vi "GUI main.vi"() -> ()   [LabVIEW 2020]
doc: "Use this template to build a producer/consumer design pattern with events to produce queue items. Use this design pattern instead of the User Interface Event Handler pattern for user interfaces when you want to execute code asynchronously in response to an event without slowing the user interface responsiveness."
uses:
  General PJVS driver/Type definitions/PJVS Type.ctl
  General PJVS driver/QPSsettings.ctl
  Measurement/Type definitions/Measuement properties.ctl
  Measurement/Type definitions/Measurement ID.ctl
  Measurement/Type definitions/Trigger mode.ctl
  General PJVS driver/Type definitions/PJVS Setup.ctl
  PJVS drivers/acsvcontrol-driver/build/ACSVcontrol-driver_0.2.0.0.llb/Timeouts.ctl
  PJVS drivers/JV modified NPL Bias source/DataSocketCluster external.ctl
  external libraries/AWG/AWG Session.ctl
  external libraries/AWG/AWG Type.ctl
  external libraries/AWG/CMI Clock Divider v2/CMI ckd2 Session.ctl
  external libraries/AWG/CMI Clock Divider v2/CMI ckd2 Source Mode.ctl
  external libraries/AWG/CMI Clock Divider v2/CMI ckd2 Divisor Mode.ctl
  external libraries/AWG/CMI Sync V3/CMI Sync V3 session.ctl
  external libraries/AWG/CMI Sync V3/Configure/CMI Sync V3 Reference Clock Source.ctl
  external libraries/AWG/CMI Sync V3/Configure/CMI Sync V3 HV input Range.ctl
  external libraries/AWG/CMI Sync V3/Configure/CMI Sync V3 Trigger Input Level.ctl
  external libraries/AWG/CMI Sync V3/Configure/CMI Sync V3 Channel 1 Mode.ctl
  external libraries/AWG/CMI Sync V3/Configure/CMI Sync V3 Channel Output Levels.ctl
  external libraries/AWG/CMI Sync V3/Configure/CMI Sync V3 Channel 2 Mode.ctl
  external libraries/AWG/CMI Sync V3/Configure/CMI Sync V3 Channel 3 Mode.ctl
  external libraries/AWG/CMI Sync V3/Configure/CMI Sync V3 Channel 1 Divisor Entry Mode.ctl
  external libraries/externals needed for AWG/ADC Trig Config.ctl
  external libraries/externals needed for AWG/ADC Trig Mode Source.ctl
  external libraries/externals needed for AWG/ADC Trig Coupling.ctl
  external libraries/externals needed for AWG/ADC Trig Slope.ctl
  external libraries/AWG/RaS HMF2500/HMF2500 Config.ctl
  <vilib>/Utility/error.llb/DialogType.ctl
  <vilib>/Utility/error.llb/Error Cluster From Error Code.vi
  <vilib>/ErrorRing/Error Ring.xnode
  external libraries/TWM client.lvlibp
  external libraries/varilib/varilib.lvlib
  PJVS drivers/acsvcontrol-driver/build/ACSVcontrol-driver_0.2.0.0.llb/ACSVcontrol-driver.lvlib
  external libraries/AWG/AWG.lvlib
  external libraries/AWG/CMI Sync V3/CMI Sync Unit V3.lvlib
panel:
  out "Measurement status":string
  in  "Setup awg":bool
  out "qps settings":T1={"TWM pipe name"="\\\\.\\pipe\\TWM:server", "meas"={"Measurement ID"=enum."1", "Description"="3 phase, 3 ADC, 1 PJVS", "Switching matrix M"=[], "Signal frequency  (Hz)"=50.0, "Signal amplitudes (V)"=[], "PRs (s)"=1.0, "PRe (s)"=10.0, "MRs (s)"=0.0, "MRe (s)"=0.0, "Set PJVS frequency (Hz)"=50.0, "PJVS reference voltages (1 period, V)"=[], "Requiested PJVS steps"=10, "Sampling f (Hz)"=0.0, "Trigger mode"=enum."Trigger every MX switch", "Timing matrix (periods)"=[], "Record length (multiples of M)"=1, "Calculated"={"Triggers to next path (line of sequence)"=[], "Record samples"=0, "Sample indexes of switches"=[], "PRs (samples)"=0, "PRe (samples)"=0, "MRs (samples)"=0, "MRe (samples)"=0, "Trigger frequency  (Hz)"=50.0, "Measurement druation (s)"=0.0}}, "PJVS setup"={"PJVS type"=enum."AC-supraVOLTcontrol", "Status Refnum"=refnum, "AC-supraVOLTcontrol"={"IP address:port (0.0.0.0:0000)"="0.0.0.0:0000", "Timeouts"={"TCP Read & Write (ms)"=7000, "Sensors readout"=5000, "PJVS setup"=10000, "Nullmeter readout"=5000, "Multiplexer setup"=3000, "57XX setup"=15000, "Generator setup"=5000, "Synthesizer setup"=3000, "Sampler readout"=10000}, "Simulation mode"=FALSE, "Debug mode"=FALSE}, "NPL bias source"={"DataSocketCluster"={"Server Machine"="CZC105BD8M", "Client Machine"="localhost", "Data"="P2", "TimeStamp"=0.0, "Count"=1, "Target Process"="General Server"}}}, "awg"={"type"=enum."Agilent 331xxA to 332xxA", "VISA"="", "enable 10MHz ref"=FALSE, "cmi ckd2"={"VISA"="", "clock source"=enum."Auto", "manual ref clk"=FALSE, "ref clock [Hz]"=0.0, "div mode"=enum."Set divisor directly"}, "cmi sync v3"={"VISA"="", "baud rate [bd/s]"=115200, "source"=enum."Auto", "hv range"=enum."1kV", "fsrc is fixed"=FALSE, "fsrc [Hz]"=10000000.0, "freq integ [s]"=1.0, "freq filter"=5, "trig level"=enum."TTL 5V", "chn1 mode"=enum."Source divider", "chn1 level"=enum."Positive 5V", "chn2 mode"=enum."Source divider", "chn2 level"=enum."Positive 5V", "chn2 div"=1, "chn3 mode"=enum."Chn 1 Active", "chn3 level"=enum."Positive 5V", "chn1 div entry"=enum."Calculate nearest divisor from measured fx", "chn1 dev limit [%]"=1.0, "chn1 check dev"=FALSE}, "trigger"={"source"=enum."Immediate", "level [V]"=0.0, "coupling"=enum."DC", "slope"=enum."POS"}, "HMF2500 cfg"={"Baud Rate"=9600, "Parity"=0, "Data Bits"=8, "Flow Control"=4}}, "Measurement status Ref"=refnum, "TWM status Ref"=refnum, "Abort Ref"=refnum} {"awg"."HMF2500 cfg"."Flow Control" items=["None", "XON/XOFF", "RTS/CTS", "XON/XOFF & RTS/CTS", "DTR/DSR", "XON/XOFF & DTR/DSR"]; "awg"."HMF2500 cfg"."Data Bits" items=["7"=7, "8"=8]; "awg"."HMF2500 cfg"."Parity" items=["None", "Odd", "Even", "Mark", "Space"]; "awg"."HMF2500 cfg"."Baud Rate" items=["300"=300, "600"=600, "1200"=1200, "2400"=2400, "4800"=4800, "9600"=9600, "19200"=19200]; "awg"."cmi sync v3"."chn2 div" min=1 max=100000000 step=1; "awg"."cmi sync v3"."fsrc [Hz]" format="%_8p"; "PJVS setup"."NPL bias source"."DataSocketCluster"."TimeStamp" format="%.2f"; "meas"."Calculated"."Trigger frequency  (Hz)" format="%#_6p"; "meas"."Record length (multiples of M)" min=1 step=1; "meas"."PJVS reference voltages (1 period, V)" format="%.9g"; "meas"."MRe (s)" format="%#_4p"; "meas"."MRs (s)" format="%#_4p"; "meas"."PRe (s)" format="%#.4p"; "meas"."PRs (s)" format="%#_4p"}
  in  "Measure":bool
  out "gui_unlock_for_measure":refnum<vi>[](array[refnum])
  out "gui_to_lock":refnum<vi>[](array[refnum])
  out "Measurement description":string
  in  "Setup meas":bool
  in  "Abort":bool
  out "PJVS status":string
  out "TWM Status":string
  out "PJVS":T6
  in  "Test TWM":bool
  in  "TWM pipe name":string="\\\\.\\pipe\\TWM:server"
  in  "About":bool
  in  "Setup pjvs":bool
  in  "Quit":bool
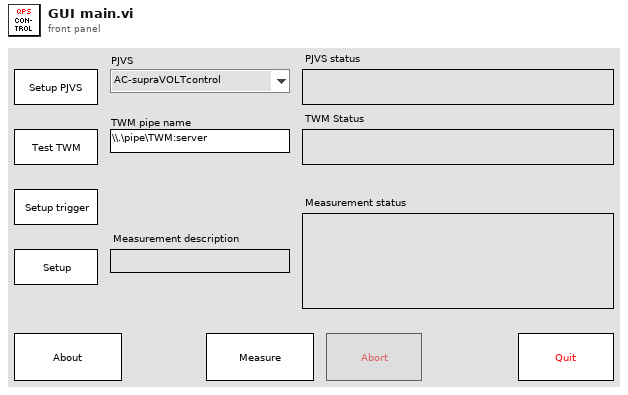
[diagram p1: front panel]
types:
  T1 = typedef "QPSsettings.ctl" = cluster{"TWM pipe name":string, "meas":T2, "PJVS setup":T5, "awg":T9, "Measurement status Ref":refnum<vi>, "TWM status Ref":refnum<vi>, "Abort Ref":refnum<vi>}
  T2 = typedef "Measuement properties.ctl" = cluster{"Measurement ID":T3, "Description":string, "Switching matrix M":u32[][], "Signal frequency  (Hz)":dbl, "Signal amplitudes (V)":dbl[], "PRs (s)":dbl, "PRe (s)":dbl, "MRs (s)":dbl, "MRe (s)":dbl, "Set PJVS frequency (Hz)":dbl, "PJVS reference voltages (1 period, V)":dbl[], "Requiested PJVS steps":u32, "Sampling f (Hz)":dbl, "Trigger mode":T4, "Timing matrix (periods)":i32[], "Record length (multiples of M)":u32, "Calculated":cluster{"Triggers to next path (line of sequence)":u32[], "Record samples":u32, "Sample indexes of switches":u32[], "PRs (samples)":i32, "PRe (samples)":i32, "MRs (samples)":i32, "MRe (samples)":i32, "Trigger frequency  (Hz)":dbl, "Measurement druation (s)":dbl}}
  T3 = typedef "Measurement ID.ctl" = enum16{"M", "1", "2", "3"}
  T4 = typedef "Trigger mode.ctl" = enum16{"Trigger every MX switch", "Trigger every sample"}
  T5 = typedef "PJVS Setup.ctl" = cluster{"PJVS type":T6, "Status Refnum":refnum<vi>, "AC-supraVOLTcontrol":cluster{"IP address:port (0.0.0.0:0000)":string, "Timeouts":T7, "Simulation mode":bool, "Debug mode":bool}, "NPL bias source":cluster{"DataSocketCluster":T8}}
  T6 = typedef "PJVS Type.ctl" = enum16{"AC-supraVOLTcontrol", "JV modified NPL bias control"}
  T7 = typedef "ACSVcontrol-driver.lvlib/Timeouts.ctl" = cluster{"TCP Read & Write (ms)":i32, "Sensors readout":i32, "PJVS setup":i32, "Nullmeter readout":i32, "Multiplexer setup":i32, "57XX setup":i32, "Generator setup":i32, "Synthesizer setup":i32, "Sampler readout":i32}
  T8 = typedef "DataSocketCluster external.ctl" = cluster{"Server Machine":string, "Client Machine":string, "Data":string, "TimeStamp":dbl, "Count":i32, "Target Process":string}
  T9 = typedef "AWG.lvlib/AWG Session.ctl" = cluster{"type":T10, "VISA":refnum<visa-resource-name>, "enable 10MHz ref":bool, "cmi ckd2":T11, "cmi sync v3":T14, "trigger":T23, "HMF2500 cfg":T27}
  T10 = typedef "AWG.lvlib/AWG Type.ctl" = enum16{"Agilent 331xxA to 332xxA", "Agilent 335xxA to 336xxA", "Tektronix AFG3101C", "R&S HMF25xx", "CMI Clock Divider v2", "CMI Sync Unit V3", "dummy"}
  T11 = typedef "AWG.lvlib/CMI ckd2 Session.ctl" = cluster{"VISA":refnum<visa-resource-name>, "clock source":T12, "manual ref clk":bool, "ref clock [Hz]":dbl, "div mode":T13}
  T12 = typedef "AWG.lvlib/CMI ckd2 Source Mode.ctl" = enum16{"Auto", "LF clock", "HF clock", "Internal"}
  T13 = typedef "AWG.lvlib/CMI ckd2 Divisor Mode.ctl" = enum16{"Set divisor directly", "Set divisor by frequency"}
  T14 = typedef "AWG.lvlib/CMI Sync Unit V3.lvlib/CMI Sync V3 session.ctl" = cluster{"VISA":refnum<visa-resource-name>, "baud rate [bd/s]":i32, "source":T15, "hv range":T16, "fsrc is fixed":bool, "fsrc [Hz]":dbl, "freq integ [s]":dbl, "freq filter":i32, "trig level":T17, "chn1 mode":T18, "chn1 level":T19, "chn2 mode":T20, "chn2 level":T19, "chn2 div":i32, "chn3 mode":T21, "chn3 level":T19, "chn1 div entry":T22, "chn1 dev limit [%]":dbl, "chn1 check dev":bool}
  T15 = typedef "AWG.lvlib/CMI Sync Unit V3.lvlib/CMI Sync V3 Reference Clock Source.ctl" = enum16{"Auto", "Internal", "Logic", "Sine", "HV"}
  T16 = typedef "AWG.lvlib/CMI Sync Unit V3.lvlib/CMI Sync V3 HV input Range.ctl" = enum16{"10V", "60V", "250V", "1kV"}
  T17 = typedef "AWG.lvlib/CMI Sync Unit V3.lvlib/CMI Sync V3 Trigger Input Level.ctl" = enum16{"LVCMOS 3V3", "TTL 5V"}
  T18 = typedef "AWG.lvlib/CMI Sync Unit V3.lvlib/CMI Sync V3 Channel 1 Mode.ctl" = enum16{"Source divider", "DDS absolute", "DDS ratio", "DDS ratio M/N"}
  T19 = typedef "AWG.lvlib/CMI Sync Unit V3.lvlib/CMI Sync V3 Channel Output Levels.ctl" = enum16{"Positive 3V3", "Negative 3V3", "Positive 5V", "Negative 5V"}
  T20 = typedef "AWG.lvlib/CMI Sync Unit V3.lvlib/CMI Sync V3 Channel 2 Mode.ctl" = enum16{"Source divider", "Chn 1 divide"}
  T21 = typedef "AWG.lvlib/CMI Sync Unit V3.lvlib/CMI Sync V3 Channel 3 Mode.ctl" = enum16{"Chn 1 Active", "Chn 2 Active", "Chn 1 Trigger", "Chn 2 Trigger", "Gate", "PPS", "10MHz"}
  T22 = typedef "AWG.lvlib/CMI Sync Unit V3.lvlib/CMI Sync V3 Channel 1 Divisor Entry Mode.ctl" = enum16{"Set divisor directly", "Calculate nearest divisor from measured fx"}
  T23 = typedef "ADC Trig Config.ctl" = cluster{"source":T24, "level [V]":dbl, "coupling":T25, "slope":T26}
  T24 = typedef "ADC Trig Mode Source.ctl" = enum16{"Immediate", "External", "Level"}
  T25 = typedef "ADC Trig Coupling.ctl" = enum16{"DC", "AC"}
  T26 = typedef "ADC Trig Slope.ctl" = enum16{"POS", "NEG"}
  T27 = typedef "AWG.lvlib/HMF2500 Config.ctl" = cluster{"Baud Rate":u32, "Parity":u16, "Data Bits":u16, "Flow Control":u16}
  T28 = typedef "DialogType.ctl" = u16
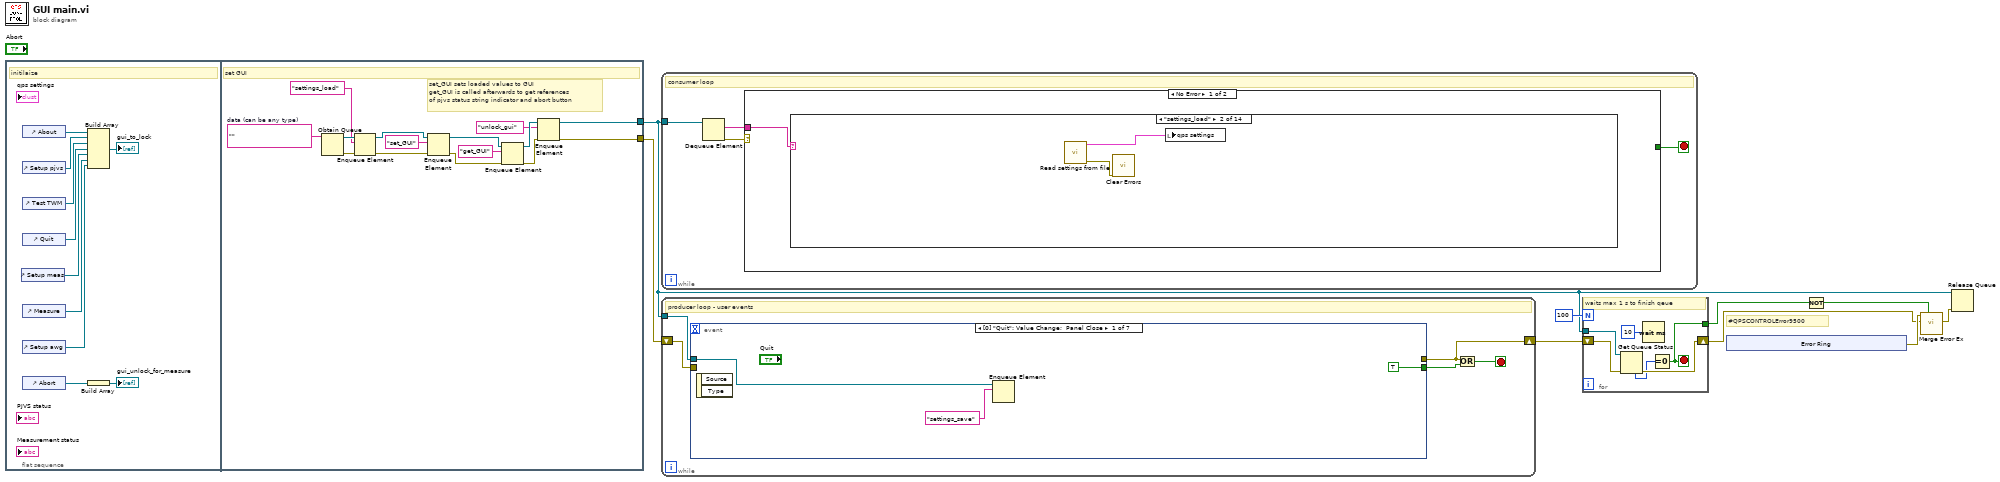
[diagram p0: block diagram]
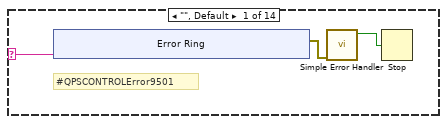
[diagram p2: hidden frame]
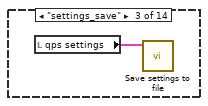
[diagram p3: hidden frame]
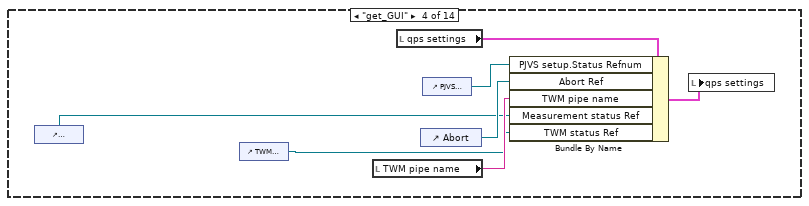
[diagram p4: hidden frame]
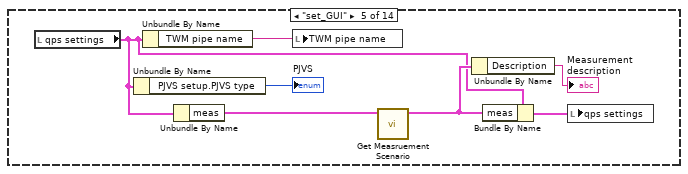
[diagram p5: hidden frame]
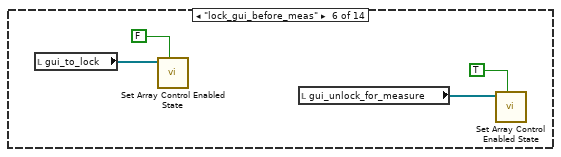
[diagram p6: hidden frame]
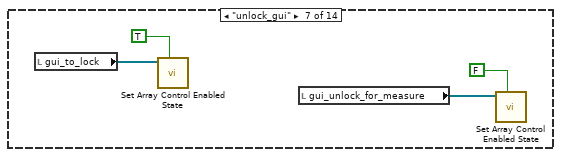
[diagram p7: hidden frame]
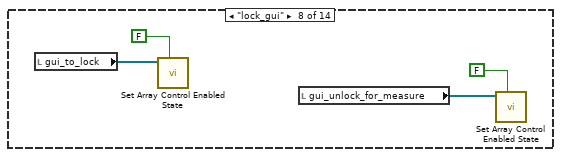
[diagram p8: hidden frame]
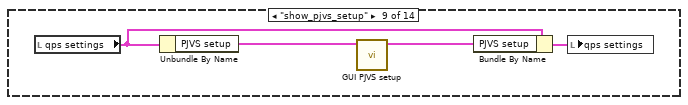
[diagram p9: hidden frame]
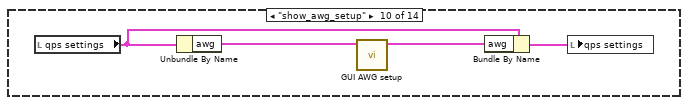
[diagram p10: hidden frame]
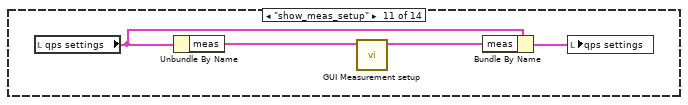
[diagram p11: hidden frame]
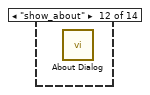
[diagram p12: hidden frame]
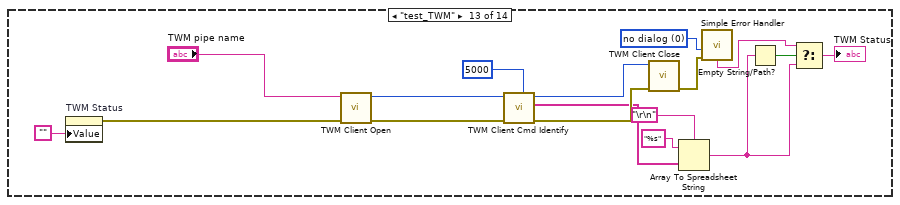
[diagram p13: hidden frame]
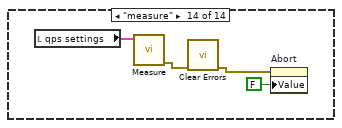
[diagram p14: hidden frame]
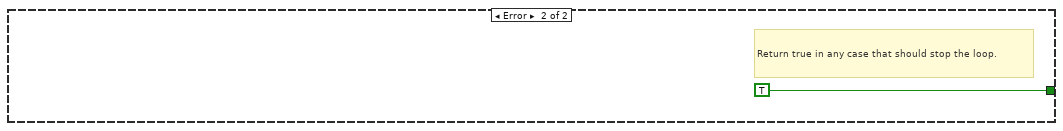
[diagram p15: hidden frame]
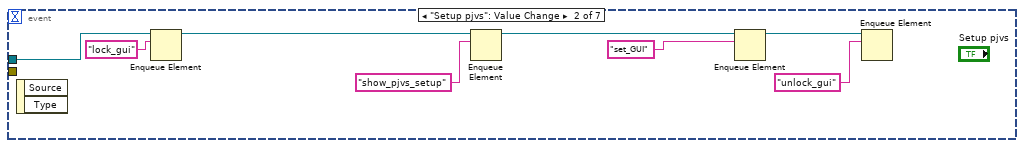
[diagram p16: hidden frame]
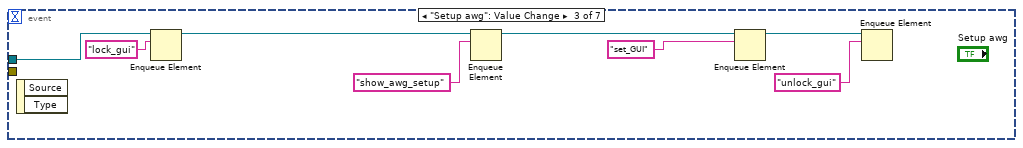
[diagram p17: hidden frame]
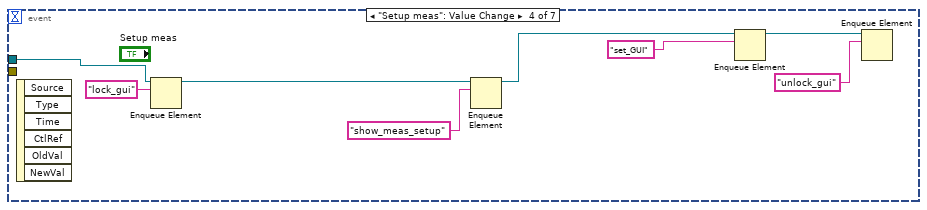
[diagram p18: hidden frame]
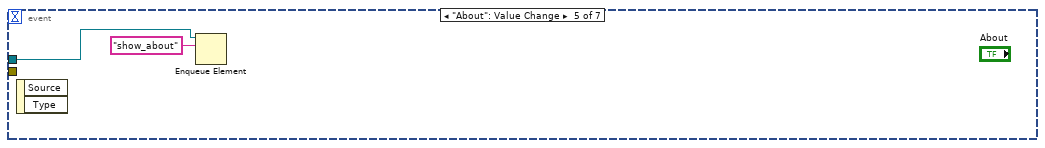
[diagram p19: hidden frame]
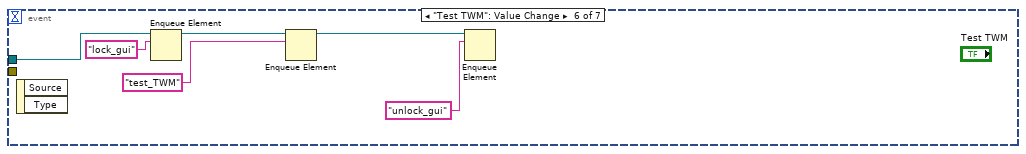
[diagram p20: hidden frame]
diagram:
  # "#QPSCONTROLError9500"
  n1 = flat-sequence {
    tunnel: [w24] -> w3
    tunnel: [w21] -> w9
    frame #0 {
      # "initilaize"
      n2 = control-ref of="Setup meas"() -> (w16:refnum<vi>)
      n3 = control-ref of="About"() -> (w12:refnum<vi>)
      n4 = control-ref of="Setup pjvs"() -> (w13:refnum<vi>)
      n5 = control-ref of="Test TWM"() -> (w14:refnum<vi>)
      n6 = control-ref of="Quit"() -> (w15:refnum<vi>)
      n7 = control-ref of="Measure"() -> (w11:refnum<vi>)
      n8 = control-ref of="Setup awg"() -> (w10:refnum<vi>)
      n9 = control-ref of="Abort"() -> (w17:refnum<vi>)
      n10 = Build Array(w12, w13, w14, w15, w16, w11, w10) -> (→"gui_to_lock":refnum<vi>[])
      n11 = Build Array(w17) -> (→"gui_unlock_for_measure":refnum<vi>[])
    }
    frame #1 {
      w34 = ""  # data (can be any type)
      # "set_GUI sets loaded values to GUI\nget_GUI is called afterwards to get references\nof pjvs status string indicator and abort button"
      # "set GUI"
      n12 = Obtain Queue(element data type=w34) -> (queue out=w33:refnum<queue>, error out=w32:errorcluster)  [unwired: 4 in, 1 out]
      n13 = Enqueue Element(queue=w33, element="settings_load", error in (no error)=w32) -> (queue out=w26:refnum<queue>, error out=w29:errorcluster)  [unwired: 1 in, 1 out]
      n14 = Enqueue Element(queue=w26, element="set_GUI", error in (no error)=w29) -> (queue out=w27:refnum<queue>, error out=w28:errorcluster)  [unwired: 1 in, 1 out]
      n15 = Enqueue Element(queue=w27, element="get_GUI", error in (no error)=w28) -> (queue out=w22:refnum<queue>, error out=w23:errorcluster)  [unwired: 1 in, 1 out]
      n16 = Enqueue Element(queue=w22, element="unlock_gui", error in (no error)=w23) -> (queue out=w24:refnum<queue>, error out=w21:errorcluster)  [unwired: 1 in, 1 out]
    }
  }
  n17 = while {
    tunnel: w3 -> [w38]
    stop <- w35 stop-if-true
    # "consumer loop"
    n18 = Dequeue Element(queue=w38) -> (element=w36:string, error out=w37:errorcluster)  [unwired: 2 in, 2 out]
    n19 = case shown="No Error" w37 {
      tunnel: w36 -> [w39 _]
      tunnel: [_ TRUE] -> w35
      frame No Error {
        n20 = case shown="\"settings_load\"" w39 {
          selector: w39 -> [w40 _ _ _ _ _ _ _ _ _ _ _ _ _]
          frame "", Default {
            # "#QPSCONTROLError9501"
            n21 = xnode "Error Ring"("parameter 0"=w40) -> ("error out"=w42:errorcluster)
            n22 = call <vilib>:"Simple Error Handler.vi"("error in (no error)"=w42) -> ("error?"=w41:bool)  [unwired: 4 in, 4 out]
            n23 = Stop(stop? (T)=w41) -> ()
          }
          frame "settings_load" {
            n24 = call "Read settings from file.vi"() -> ("error out"=w50:errorcluster, "QPS settings out"=w51:T1)  [unwired: 10 in]
            n25 = call <vilib>:"Clear Errors.vi"("error in (no error)"=w50) -> ()  [unwired: 5 in, 2 out]
            n26 = local write "qps settings"(w51) -> ()
          }
          frame "settings_save" {
            n27 = local read "qps settings"() -> (w52:T1)
            n28 = call "Save settings to file.vi"("QPS settings"=w52) -> ()  [unwired: 10 in, 1 out]
          }
          frame "get_GUI" {
            n29 = control-ref of="Measurement status"() -> (w54:refnum<vi>)
            n30 = control-ref of="TWM Status"() -> (w53:refnum<vi>)
            n31 = local read "TWM pipe name"() -> (w55:string)
            n32 = local read "qps settings"() -> (w59:T1)
            n33 = control-ref of="Abort"() -> (w57:refnum<vi>)
            n34 = control-ref of="PJVS status"() -> (w56:refnum<vi>)
            n35 = Bundle By Name(cluster=w59, "PJVS setup.Status Refnum"=w56, "Abort Ref"=w57, "TWM pipe name"=w55, "Measurement status Ref"=w54, "TWM status Ref"=w53) -> (w58:T1)
            n36 = local write "qps settings"(w58) -> ()
          }
          frame "set_GUI" {
            n37 = local read "qps settings"() -> (w61:T1)
            n38 = Unbundle By Name(w61) -> ("PJVS setup.PJVS type"=→"PJVS":T6)
            n39 = Unbundle By Name(w61) -> ("TWM pipe name"=w60:string)
            n40 = Unbundle By Name(w61) -> ("meas"=w64:T2)
            n41 = local write "TWM pipe name"(w60) -> ()
            n42 = call "Get Measruement Scenario.vi"("Measurement properties"=w64) -> ("Measurement properties out"=w63:T2)  [unwired: 10 in]
            n43 = Unbundle By Name(w63) -> ("Description"=→"Measurement description":string)
            n44 = Bundle By Name(cluster=w61, "meas"=w63) -> (w62:T1)
            n45 = local write "qps settings"(w62) -> ()
          }
          frame "lock_gui_before_meas" {
            n46 = local read "gui_to_lock"() -> (w70:refnum<vi>[])
            n47 = call "Set Array Control Enabled State.vi"("enabled (T)"=FALSE, "reference array in"=w70) -> ()  [unwired: 8 in, 2 out]
            n48 = local read "gui_unlock_for_measure"() -> (w68:refnum<vi>[])
            n49 = call "Set Array Control Enabled State.vi"("enabled (T)"=TRUE, "reference array in"=w68) -> ()  [unwired: 8 in, 2 out]
          }
          frame "unlock_gui" {
            n50 = local read "gui_to_lock"() -> (w74:refnum<vi>[])
            n51 = call "Set Array Control Enabled State.vi"("enabled (T)"=TRUE, "reference array in"=w74) -> ()  [unwired: 8 in, 2 out]
            n52 = local read "gui_unlock_for_measure"() -> (w73:refnum<vi>[])
            n53 = call "Set Array Control Enabled State.vi"("enabled (T)"=FALSE, "reference array in"=w73) -> ()  [unwired: 8 in, 2 out]
          }
          frame "lock_gui" {
            n54 = local read "gui_to_lock"() -> (w78:refnum<vi>[])
            n55 = call "Set Array Control Enabled State.vi"("enabled (T)"=FALSE, "reference array in"=w78) -> ()  [unwired: 8 in, 2 out]
            n56 = local read "gui_unlock_for_measure"() -> (w77:refnum<vi>[])
            n57 = call "Set Array Control Enabled State.vi"("enabled (T)"=FALSE, "reference array in"=w77) -> ()  [unwired: 8 in, 2 out]
          }
          frame "show_pjvs_setup" {
            n58 = local read "qps settings"() -> (w81:T1)
            n59 = Unbundle By Name(w81) -> ("PJVS setup"=w82:T5)
            n60 = call "GUI PJVS setup.vi"("PJVS setup"=w82) -> ("PJVS setup out"=w80:T5)  [unwired: 10 in]
            n61 = Bundle By Name(cluster=w81, "PJVS setup"=w80) -> (w79:T1)
            n62 = local write "qps settings"(w79) -> ()
          }
          frame "show_awg_setup" {
            n63 = local read "qps settings"() -> (w86:T1)
            n64 = Unbundle By Name(w86) -> ("awg"=w84:T9)
            n65 = call "GUI AWG setup.vi"("awg session"=w84) -> ("awg session out"=w83:T9)  [unwired: 10 in]
            n66 = Bundle By Name(cluster=w86, "awg"=w83) -> (w85:T1)
            n67 = local write "qps settings"(w85) -> ()
          }
          frame "show_meas_setup" {
            n68 = local read "qps settings"() -> (w90:T1)
            n69 = Unbundle By Name(w90) -> ("meas"=w88:T2)
            n70 = call "GUI Measurement setup.vi"("Measurement properties"=w88) -> ("Measurement properties out"=w87:T2)  [unwired: 10 in]
            n71 = Bundle By Name(cluster=w90, "meas"=w87) -> (w89:T1)
            n72 = local write "qps settings"(w89) -> ()
          }
          frame "show_about" {
            n73 = call "About Dialog.vi"() -> ()  [unwired: 12 in]
          }
          frame "test_TWM" {
            w95 = T28 0 items=["no dialog", "OK message", "continue or stop message", "OK message + warnings", "continue/stop + warnings"] ("type of dialog (OK msg:1)")
            n74 = property on="TWM Status" class="Str"("Value"="") -> (error out=w98:errorcluster)  [unwired: 2 in, 1 out]
            n75 = call "TWM Client Open.vi"("error in"=w98, "pipe name"="TWM pipe name") -> ("error out"=w106:errorcluster, "handle out"=w104:i32)  [unwired: 8 in]
            n76 = call "TWM Client Cmd Identify.vi"("timeout [ms]"=5000, "error in"=w106, "handle"=w104) -> ("error out"=w107:errorcluster, "channel idns"=w101:string[], "handle out"=w103:i32)  [unwired: 5 in, 1 out]
            n77 = call "TWM Client Close.vi"("error in"=w107, "handle in"=w103) -> ("error out"=w96:errorcluster)  [unwired: 9 in]
            n78 = Array To Spreadsheet String(delimiter (Tab)="\r\n", array=w101, 3:"%s" ("format string")) -> (spreadsheet string=w92:string)
            n79 = call <vilib>:"Simple Error Handler.vi"("type of dialog (OK msg:1)"=w95, "error in (no error)"=w96) -> ("message"=w93:string)  [unwired: 3 in, 4 out]
            n80 = Empty String/Path?(string/path=w92) -> (empty?=w94:bool)
            n81 = Select(t=w93, s=w94, f=w92) -> (s? t:f=→"TWM Status":string)
          }
          frame "measure" {
            n82 = local read "qps settings"() -> (w111:T1)
            n83 = call "Measure.vi"("QPS settings"=w111) -> ("error out"=w110:errorcluster)  [unwired: 9 in, 1 out]
            n84 = call <vilib>:"Clear Errors.vi"("error in (no error)"=w110) -> ("error out"=w109:errorcluster)  [unwired: 5 in, 1 out]
            n85 = property on="Abort" class="Bool (strict)"(error in=w109, "Value"=FALSE ("Abort")) -> ()  [unwired: 1 in, 2 out]
          }
        }
      }
      frame Error {
        # "Return true in any case that should stop the loop."
      }
    }
  }
  n86 = while {
    shift-right: [w113] -> w1
    shift-left: w9 -> [w116]
    tunnel: w3 -> [w117]
    stop <- w114 stop-if-true
    # "producer loop - user events"
    n87 = event shown="[0] \"Quit\": Value Change;  Panel Close" {
      selector: _ -> [_ _ _ _ _ _ _]
      dyn-events: _ -> [_ _ _ _ _ _ _]
      timeout: _ -> [_ _ _ _ _ _ _]
      tunnel: w117 -> [w118 w122 w131 w139 w145 w149 w158]
      tunnel: w116 -> [_ _ _ _ _ _ _]
      tunnel: [_ _ _ _ _ _ w153] -> w113
      tunnel: [TRUE ("cancel") _ _ _ _ _ _] -> w115
      event "Quit": Value Change; Panel Close {
        n88 = event-data() -> ()  [unwired: 1 in, 2 out]
        n89 = Enqueue Element(queue=w118, element="settings_save") -> ()  [unwired: 2 in, 3 out]
      }
      event "Setup pjvs": Value Change {
        n90 = event-data() -> ()  [unwired: 1 in, 2 out]
        n91 = Enqueue Element(queue=w122, element="lock_gui") -> (queue out=w121:refnum<queue>)  [unwired: 2 in, 2 out]
        n92 = Enqueue Element(queue=w121, element="show_pjvs_setup") -> (queue out=w127:refnum<queue>)  [unwired: 2 in, 2 out]
        n93 = Enqueue Element(queue=w127, element="set_GUI") -> (queue out=w123:refnum<queue>)  [unwired: 2 in, 2 out]
        n94 = Enqueue Element(queue=w123, element="unlock_gui") -> ()  [unwired: 2 in, 3 out]
      }
      event "Setup awg": Value Change {
        n95 = event-data() -> ()  [unwired: 1 in, 2 out]
        n96 = Enqueue Element(queue=w131, element="lock_gui") -> (queue out=w130:refnum<queue>)  [unwired: 2 in, 2 out]
        n97 = Enqueue Element(queue=w130, element="show_awg_setup") -> (queue out=w135:refnum<queue>)  [unwired: 2 in, 2 out]
        n98 = Enqueue Element(queue=w135, element="set_GUI") -> (queue out=w129:refnum<queue>)  [unwired: 2 in, 2 out]
        n99 = Enqueue Element(queue=w129, element="unlock_gui") -> ()  [unwired: 2 in, 3 out]
      }
      event "Setup meas": Value Change {
        n100 = event-data() -> ()  [unwired: 1 in, 6 out]
        n101 = Enqueue Element(queue=w139, element="lock_gui") -> (queue out=w138:refnum<queue>)  [unwired: 2 in, 2 out]
        n102 = Enqueue Element(queue=w138, element="show_meas_setup") -> (queue out=w144:refnum<queue>)  [unwired: 2 in, 2 out]
        n103 = Enqueue Element(queue=w144, element="set_GUI") -> (queue out=w137:refnum<queue>)  [unwired: 2 in, 2 out]
        n104 = Enqueue Element(queue=w137, element="unlock_gui") -> ()  [unwired: 2 in, 3 out]
      }
      event "About": Value Change {
        n105 = event-data() -> ()  [unwired: 1 in, 2 out]
        n106 = Enqueue Element(queue=w145, element="show_about") -> ()  [unwired: 2 in, 3 out]
      }
      event "Test TWM": Value Change {
        n107 = event-data() -> ()  [unwired: 1 in, 2 out]
        n108 = Enqueue Element(queue=w149, element="lock_gui") -> (queue out=w148:refnum<queue>)  [unwired: 2 in, 2 out]
        n109 = Enqueue Element(queue=w148, element="test_TWM") -> (queue out=w147:refnum<queue>)  [unwired: 2 in, 2 out]
        n110 = Enqueue Element(queue=w147, element="unlock_gui") -> ()  [unwired: 2 in, 3 out]
      }
      event "Measure": Value Change {
        n111 = event-data() -> ()  [unwired: 1 in, 6 out]
        n112 = Enqueue Element(queue=w158, element="lock_gui_before_meas") -> (queue out=w157:refnum<queue>)  [unwired: 2 in, 2 out]
        n113 = Enqueue Element(queue=w157, element="measure") -> (queue out=w156:refnum<queue>)  [unwired: 2 in, 2 out]
        n114 = Enqueue Element(queue=w156, element="unlock_gui") -> (error out=w153:errorcluster)  [unwired: 2 in, 2 out]
      }
    }
    n115 = Or(x=w113, y=w115) -> (x .or. y?=w114:bool)
  }
  n116 = for {
    N: 100 -> [_]
    tunnel: w3 -> [w165]
    shift-right: [w163] -> w7
    shift-left: w1 -> [w164]
    tunnel: [w160] -> w5
    stop <- w160 stop-if-true
    # "waits max 1 s to finish qeue"
    n117 = Get Queue Status(queue=w165, error in (no error)=w164) -> (error out=w163:errorcluster, # elements in queue=w161:i32)  [unwired: 1 in, 6 out]
    n118 = Wait (ms)(milliseconds to wait=u32 10) -> ()  [unwired: 1 out]
    n119 = Equal To 0?(x=w161) -> (x = 0?=w160:bool)
  }
  n120 = xnode "Error Ring"() -> ("error out"=w8:errorcluster)
  n121 = Not(x=w5) -> (.not. x?=w6:bool)
  n122 = call "Merge Error Ex.vi"("Is error? (False)"=w6, "main error in (no error)"=w7, "second error in"=w8) -> ("error out"=w2:errorcluster)  [unwired: 8 in]
  n123 = Release Queue(queue=w3, error in (no error)=w2) -> ()  [unwired: 1 in, 3 out]
